vi "RT_Moment_of_Inertia_in_DLR_Navigation_Reference_System(SubVI).vi"(10 "i":i32, 11 "Data":dbl[][](array[numeric])) -> (3 "I (kg.m^2)":dbl[][](array[numeric]))   [LabVIEW 2017]
uses:
  <vilib>/Analysis/Matrix/Datatypes/RealMatrix.ctl
  <vilib>/Analysis/Matrix/Numeric/Conversions/Matrix To Array - RM.vi
  <vilib>/Analysis/NI_AALBase.lvlib
  <vilib>/Analysis/baseanly.llb/Real A x B.vi
  <vilib>/Analysis/Matrix/NI_Matrix.lvlib
  <vilib>/Analysis/Matrix/Numeric/Conversions/Array To Matrix - RA2.vi
panel:
  out "I_b_matrix (kg.m^2)":T1
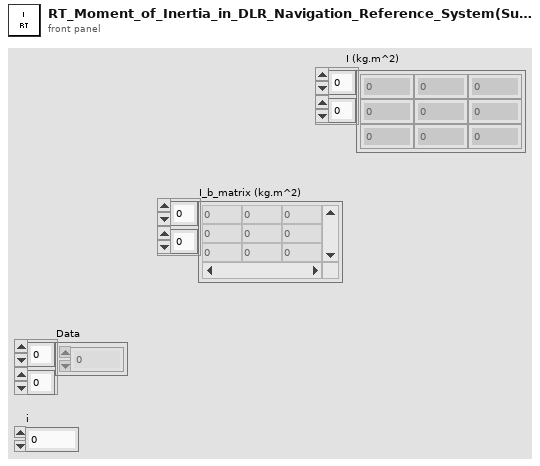
[diagram p1: front panel]
types:
  T1 = typedef "NI_Matrix.lvlib/RealMatrix.ctl" = dbl[][]
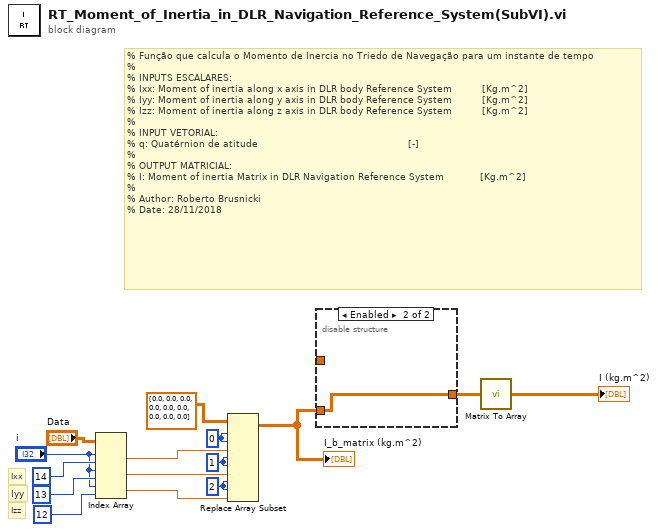
[diagram p0: block diagram]
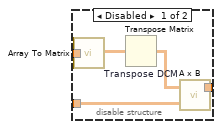
[diagram p2: hidden frame]
diagram:
  w2 = 2 ("index (col)")
  w3 = 1 ("index (row)")
  w5 = 0 ("index (col)")
  # "Izz"
  # "Iyy"
  # "Ixx"
  # "% Função que calcula o Momento de Inercia no Triedo de Navegação para um instante de tempo\n%\n% INPUTS ESCALARES:\n% Ixx: Moment of inertia along x axis in DLR body Reference System          [Kg.m^2]\n% Iyy: Moment of inertia along y axis in DLR body Reference System          [Kg.m^2]\n% Izz: Moment of inertia along z axis in DLR body Reference System          [Kg.m^2]\n% \n% INPUT VETORIAL:\n% q: Quatérnion de atitude                                                  [-]\n%\n% OUTPUT MATRICIAL:\n% I: Moment of inertia Matrix in DLR Navigation Reference System            [Kg.m^2]\n%\n% Author: Roberto Brusnicki\n% Date: 28/11/2018"
  n1 = Index Array(array="Data", index (row) #1="i", index (col) #1=14 ("disabled index (col)"), index (row) #2="i", index (col) #2=13 ("disabled index (col)"), index (row) #3="i", index (col) #3=12 ("disabled index (col)")) -> (element #1=w12:dbl, element #2=w13:dbl, element #3=w14:dbl)
  n2 = Replace Array Subset(array=T1 [[0.0, 0.0, 0.0], [0.0, 0.0, 0.0], [0.0, 0.0, 0.0]] ("transposed matrix"), new element #1=w12, index (row) #1=w5, index (col) #1=w5, new element #2=w13, index (row) #2=w3, index (col) #2=w3, new element #3=w14, index (row) #3=w2, index (col) #3=w2) -> (w15:T1)
  "I_b_matrix (kg.m^2)" <- w15
  n3 = disable-structure shown="Enabled" {
    disable-tunnel: w15 -> [w20 w21]
    disable-tunnel: _ -> [w17 _]
    disable-tunnel: [w16 w21] -> w11
    frame Disabled {
      n4 = call-poly <vilib>:"Array To Matrix.vi"("Real 2D Array"=w17) -> ("Real Matrix"=w18:T1)
      n5 = Transpose Matrix "Transpose DCM"(1:w18) -> (0:w19:T1)
      n6 = call-poly <vilib>:"A x B.vi"("B"=w20, "A"=w19) -> ("A x B"=w16:T1)  [unwired: 1 out]
    }
    frame Enabled {
    }
  }
  n7 = call-poly <vilib>:"Matrix To Array.vi"("Real Matrix"=w11) -> ("Real 2D Array"=→"I (kg.m^2)":dbl[][])
